vi "Get Domain.vi"(8 "error in (no error)":errorcluster, 11 "Domain in":refnum<class "NI_Domain.lvclass">) -> (0 "error out":errorcluster, 2 "domain":variant, 3 "Domain out":refnum<class "NI_Domain.lvclass">)   [LabVIEW 2017, in "NI_PDE.lvlib" / "NI_Domain.lvclass"]
uses:
  <vilib>/gmath/pde.llb/DomainClass/NI_Domain.lvclass
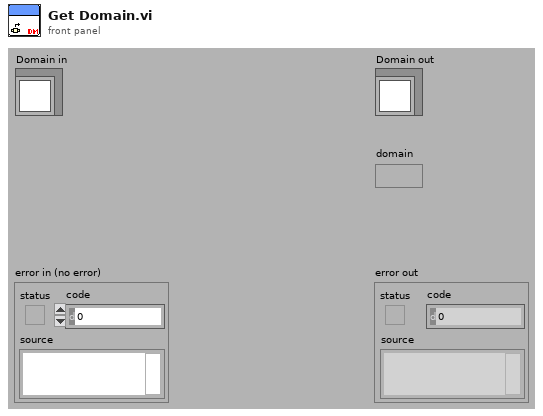
[diagram p1: front panel]
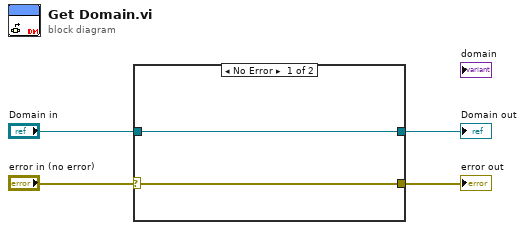
[diagram p0: block diagram]
diagram:
  n1 = case shown="No Error" "error in (no error)" {
    selector: "error in (no error)" -> [w5 w8]
    tunnel: "Domain in" -> [w6 w7]
    tunnel: [w6 w7] -> w4
    tunnel: [w5 w8] -> w3
    frame No Error {
    }
    frame Error {
    }
  }
  "Domain out" <- w4
  "error out" <- w3
